vi "Read States.vi"(8 "error in (no error)":errorcluster, 11 "ReceivePassInFuturePointTactic in":refnum<class "ReceivePassInFuturePointTactic.lvclass">) -> (0 "error out":errorcluster, 2 "States":enum16{"Exit", "Halt", "GoTo"}(ring), 3 "ReceivePassInFuturePointTactic out":refnum<class "ReceivePassInFuturePointTactic.lvclass">)   [LabVIEW 2023, in "ReceivePassInFuturePointTactic.lvclass"]
uses:
  ReceivePassInFuturePointTactic.lvclass
  ReceivePassInFuturePointTactic.lvclass/ReceivePassInFuturePointTactic.ctl
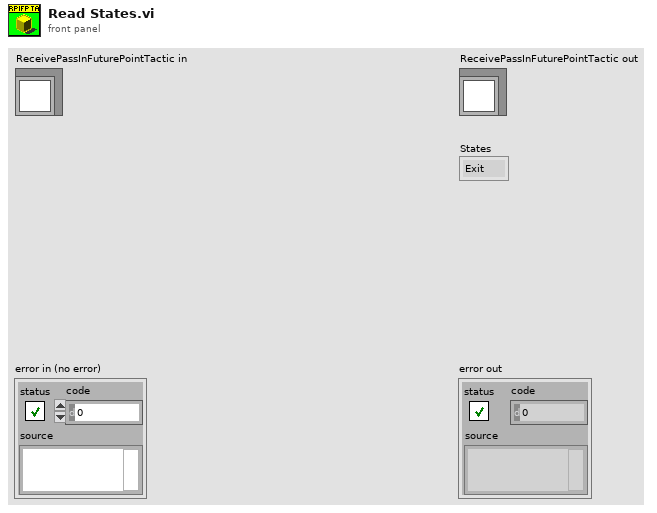
[diagram p1: front panel]
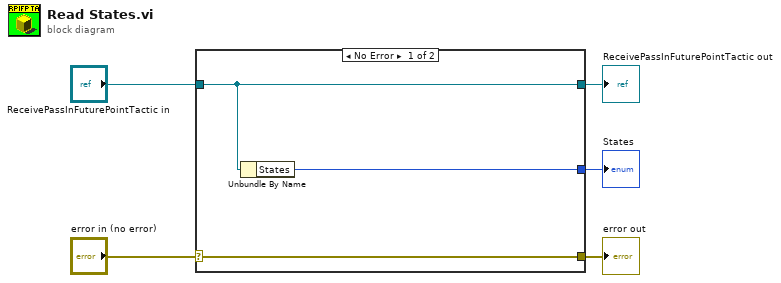
[diagram p0: block diagram]
diagram:
  n1 = case shown="No Error" "error in (no error)" {
    selector: "error in (no error)" -> [w8 w9]
    tunnel: [w8 w9] -> w4
    tunnel: [w7 w10] -> w2
    tunnel: "ReceivePassInFuturePointTactic in" -> [w7 w10]
    tunnel: [w6 _] -> w1
    frame No Error {
      n2 = Unbundle By Name(w7) -> ("States"=w6:enum16{"Exit", "Halt", "GoTo"})
    }
    frame Error {
    }
  }
  "error out" <- w4
  "ReceivePassInFuturePointTactic out" <- w2
  "States" <- w1
